vi "Lines To Words.vi"(11 "lines in":T1) -> (3 "words out":T1)   [LabVIEW 2023]
uses:
  <extravilib>/ChannelInstances/Stream-str/)Channel.ctl
  <extravilib>/ChannelInstances/Stream-str/Read With Abort.vi
  <extravilib>/ChannelInstances/Stream-str/Write With Abort.vi
  <extravilib>/ChannelInstances/Stream-str/EndpointRead.vi
  <extravilib>/ChannelInstances/Stream-str/Endpoint.vi
  <extravilib>/ChannelInstances/Stream-str/)Channel.vi
  <resource>/ChannelSupport/_ChannelSupport/WaitIfNeeded.vi
  <extravilib>/ChannelInstances/Stream-str.lvlib
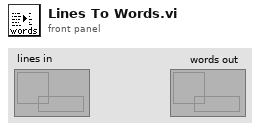
[diagram p1: front panel]
types:
  T1 = typedef "Stream-str.lvlib/)Channel.ctl" = refnum<queue>
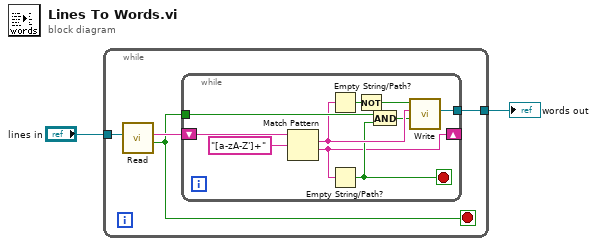
[diagram p0: block diagram]
diagram:
  n1 = while {
    tunnel: [w6] -> w2
    tunnel: "lines in" -> [w5]
    stop <- w3 stop-if-true
    n2 = call <extravilib>:"Read.vi"("channel"=w5) -> ("last element?"=w3:bool, "element"=w4:string)  [unwired: 6 in, 3 out]
    n3 = while {
      tunnel: [w16] -> w6
      shift-right: [w7] -> _
      shift-left: w4 -> [w14]
      tunnel: w3 -> [w13]
      stop <- w11 stop-if-true
      n4 = Match Pattern(string=w14, regular expression="[a-zA-Z']+" ("match pattern")) -> (match substring=w12:string, after substring=w7:string)  [unwired: 1 in, 2 out]
      n5 = Empty String/Path?(string/path=w12) -> (empty?=w9:bool)
      n6 = Empty String/Path?(string/path=w7) -> (empty?=w11:bool)
      n7 = Not(x=w9) -> (.not. x?=w8:bool)
      n8 = And(x=w13, y=w11) -> (x .and. y?=w10:bool)
      n9 = call <extravilib>:"Write.vi"("last element? (F)"=w10, "element"=w12, "element valid? (T)"=w8) -> ("channel"=w16:T1)  [unwired: 6 in, 2 out]
    }
  }
  "words out" <- w2
